vi "Read Output Till Settle.vi"(7 "timeout [ms]":u32, 8 "error in":errorcluster, 10 "settled for [ms]":u32, 11 "GOLPI ref. in":T1={"pipe handle"={"lv_proc.dll file path"=path "", "process instance handle"=[]}, "fast read timeout [ms]"=500, "fast read settle time [ms]"=10, "fast read to multiple [ms]"=1, "max elements per input line"=100, "slow read timeout [ms]"=500, "stdin double format specifier"="%_16e", "max elements per stdout output column"=100}) -> (0 "error out":errorcluster, 2 "read buffer":string, 3 "GOLPI ref. out":T1={"pipe handle"={"lv_proc.dll file path"=path "", "process instance handle"=[]}, "fast read timeout [ms]"=500, "fast read settle time [ms]"=10, "fast read to multiple [ms]"=1, "max elements per input line"=100, "slow read timeout [ms]"=500, "stdin double format specifier"="%_16e", "max elements per stdout output column"=100}, 5 "bytes remaining":i32)   [LabVIEW 2013, in "GOLPI library.lvlib"]
doc: "Continually reads output of GNU Octave. If no new data appears in the buffer for at least 'settled for' miliseconds, reading stops. If timeout is exceeded, returns only part of buffer and returns number of bytes remaining in the stdout (if any)."
uses:
  GOLPI library.lvlib
  Private/Type Definitions/GOLPI reference Type Def.ctl
  LV Process.lvlibp/Pipe Handle.ctl
  Private/Type Definitions/Custom Error Codes Enum Type Def.vi
  LV Process.lvlibp
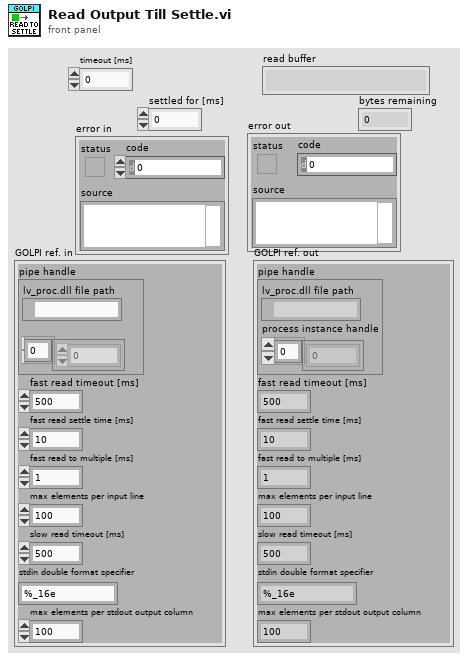
[diagram p1: front panel]
types:
  T1 = typedef "GOLPI library.lvlib/GOLPI reference Type Def.ctl" = cluster{"pipe handle":T2, "fast read timeout [ms]":u32, "fast read settle time [ms]":u32, "fast read to multiple [ms]":u32, "max elements per input line":u32, "slow read timeout [ms]":u32, "stdin double format specifier":string, "max elements per stdout output column":u32}
  T2 = typedef "LV Process.lvlibp/Pipe Handle.ctl" = cluster{"lv_proc.dll file path":path, "process instance handle":u32[]}
  T3 = typedef "GOLPI library.lvlib/Custom Error Codes Enum Type Def.vi" = enum16{"no error", "00 working directory PAR1 missing", "01 octave binary PAR1 missing", "02 octave report error PAR1", "03 empty output last cmd PAR1", "04 missing temporary file PAR1", "05 pwd PAR 1 not exist", "10 var PAR1 not string, vect", "11 var PAR1 not num, scal, ~compl", "12 var PAR1 not num, scal, compl", "13 var PAR1 not num, vect, ~compl", "14 var PAR1 not num, vect, compl", "15 var PAR1 not num, mat, ~compl", "16 var PAR1 not num, mat, ~compl", "30 WARNING read timeout", "99 not finished"}
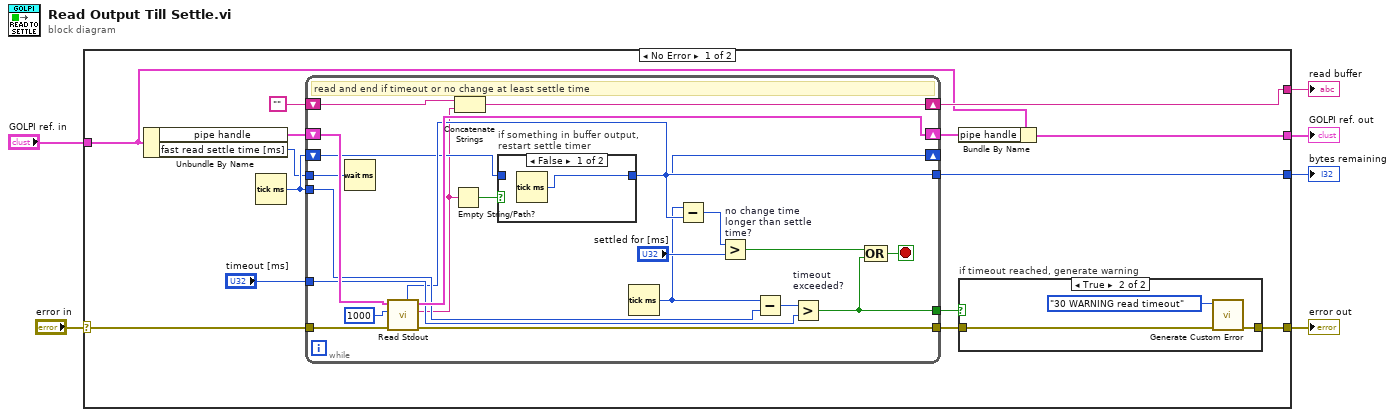
[diagram p0: block diagram]
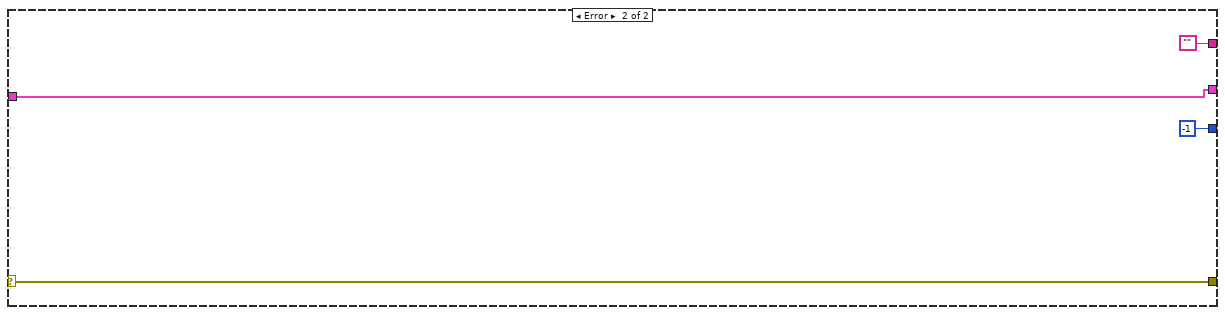
[diagram p4: hidden frame]
diagram:
  n1 = case shown="No Error" "error in" {
    selector: "error in" -> [w7 w52]
    tunnel: [w20 ""] -> w6
    tunnel: [w19 -1 ("bytes remaining")] -> w5
    tunnel: [w14 w49] -> w4
    tunnel: "GOLPI ref. in" -> [w13 w49]
    tunnel: [w8 w52] -> w2
    frame No Error {
      n2 = Unbundle By Name(w13) -> ("pipe handle"=w15:T2, "fast read settle time [ms]"=w11:u32)
      n3 = Tick Count (ms)() -> (millisecond timer value=w16:u32)
      n4 = while {
        tunnel: [w44] -> w9
        tunnel: w7 -> [w43]
        tunnel: [w38] -> w19
        shift-right: [w45] -> w12
        shift-left: w15 -> [w46]
        shift-right: [w42] -> w20
        shift-left: "" -> [w35]
        tunnel: w16 -> [w41]
        tunnel: "timeout [ms]" -> [w39]
        shift-right: [w29] -> _
        shift-left: w16 -> [w34]
        tunnel: w11 -> [w26]
        tunnel: [w25] -> w10
        stop <- w37 stop-if-true
        # "read and end if timeout or no change at least settle time"
        n5 = Wait (ms)(milliseconds to wait=w26) -> ()  [unwired: 1 out]
        n6 = call "Read Stdout.vi"("error in"=w43, "byte count"=1000, "pipe in"=w46) -> ("error out"=w44:errorcluster, "read buffer"=w30:string, "pipe out"=w45:T2, "bytes remaining"=w38:i32)  [unwired: 3 in, 2 out]
        n7 = Empty String/Path?(string/path=w30) -> (empty?=w31:bool)
        n8 = Concatenate Strings(w35, w30) -> (w42:string)
        n9 = case "if something in buffer output,\nrestart settle timer" shown="False" w31 {
          tunnel: [w47 w48] -> w29
          tunnel: w34 -> [_ w48]
          frame False {
            n10 = Tick Count (ms)() -> (millisecond timer value=w47:u32)
          }
          frame True {
          }
        }
        n11 = Tick Count (ms)() -> (millisecond timer value=w27:u32)
        n12 = Subtract(x=w27, y=w29) -> (x-y=w28:u32)
        n13 = Greater? "no change time\nlonger than settle\ntime?"(x=w28, y="settled for [ms]") -> (0:w32:bool)
        n14 = Subtract(x=w27, y=w41) -> (x-y=w40:u32)
        n15 = Greater? "timeout\nexceeded?"(x=w40, y=w39) -> (0:w25:bool)
        n16 = Compound Arithmetic op=OR(w32, w25) -> (w37:bool)
      }
      n17 = Bundle By Name(cluster=w13, "pipe handle"=w12) -> (w14:T1)
      n18 = case "if timeout reached, generate warning" shown="True" w10 {
        tunnel: [w21 w22] -> w8
        tunnel: w9 -> [w21 w23]
        frame False {
        }
        frame True {
          n19 = call "Generate Custom Error.vi"("error in"=w23, "GOLPI error"=Custom_Error_Codes_Enum_Type_Def.vi."30 WARNING read timeout") -> ("error out"=w22:errorcluster)  [unwired: 9 in]
        }
      }
    }
    frame Error {
    }
  }
  "error out" <- w2
  "read buffer" <- w6
  "bytes remaining" <- w5
  "GOLPI ref. out" <- w4
